vi "lj_read.vi"(7 "Queues":T1, 8 "error in (no error)":errorcluster, 11 "LabJackConfig":T4={"Drum Reflectors"=4, "Drum Max. Samping Window [s]"=2.0, "Drum Min. Sampling Window [s]"=0.5, "Flow Max. Samping Window [s]"=1.0, "Flow Min. Sampling Window [s]"=0.25, "Pulse value [mL]"=0.0, "RMS Sampling Window [s]"=3.0, "TC Sampling Window [s]"=0.25, "TC Scale"=[1.0, 1.0], "TC Offset [V]"=[0.0, 0.0]} {"TC Offset [V]" format="%#_f"; "TC Scale" format="%#_f"; "Pulse value [mL]" format="%#_f"}) -> (0 "error out":errorcluster, 2 "subarray":dbl[](array[numeric]), 3 "Read Data":T3 {"Peak to Peak [V]" format="%#_f"; "RMS [Hz]" format="%#_f"; "CJTemp [K]" format="%#_f"; "TC [V]" format="%#_f"; "TC [degC]" format="%#_f"; "RMS [A]" format="%#_f"; "Volume [L]" format="%#_f"; "Flow [L/min]" format="%#_f"; "Spin  [RPM]" format="%#_f"})   [LabVIEW 2025, in "LabJackEKG.lvlib"]
uses:
  LabJackEKG.lvlib
  Typedefs/AcquisitionConfig.ctl
  Typedefs/LabJackData.ctl
  Typedefs/LabJackGlobalResources.ctl
  Typedefs/CounterQueues.ctl
  Typedefs/DirectionFgvOperation.ctl
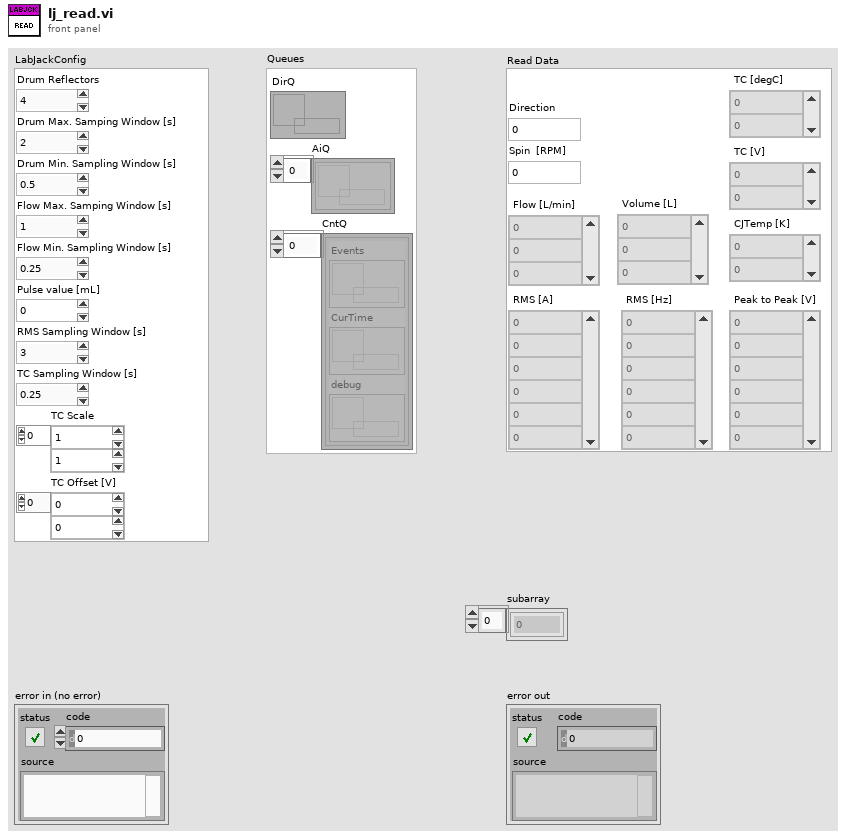
[diagram p1: front panel]
types:
  T1 = typedef "LabJackEKG.lvlib/LabJackGlobalResources.ctl" = cluster{"DirQ":refnum<queue>, "AiQ":refnum<queue>[], "CntQ":T2[]}
  T2 = typedef "LabJackEKG.lvlib/CounterQueues.ctl" = cluster{"Events":refnum<queue>, "CurTime":refnum<queue>, "debug":refnum<queue>}
  T3 = typedef "LabJackEKG.lvlib/LabJackData.ctl" = cluster{"Direction":i32, "Spin  [RPM]":dbl, "Flow [L/min]":dbl[], "Volume [L]":dbl[], "RMS [A]":dbl[], "TC [degC]":dbl[], "TC [V]":dbl[], "CJTemp [K]":dbl[], "RMS [Hz]":dbl[], "Peak to Peak [V]":dbl[]}
  T4 = typedef "LabJackEKG.lvlib/AcquisitionConfig.ctl" = cluster{"Drum Reflectors":i64, "Drum Max. Samping Window [s]":dbl, "Drum Min. Sampling Window [s]":dbl, "Flow Max. Samping Window [s]":dbl, "Flow Min. Sampling Window [s]":dbl, "Pulse value [mL]":dbl, "RMS Sampling Window [s]":dbl, "TC Sampling Window [s]":dbl, "TC Scale":dbl[], "TC Offset [V]":dbl[]}
  T5 = typedef "LabJackEKG.lvlib/DirectionFgvOperation.ctl" = enum16{"init", "process", "get"}
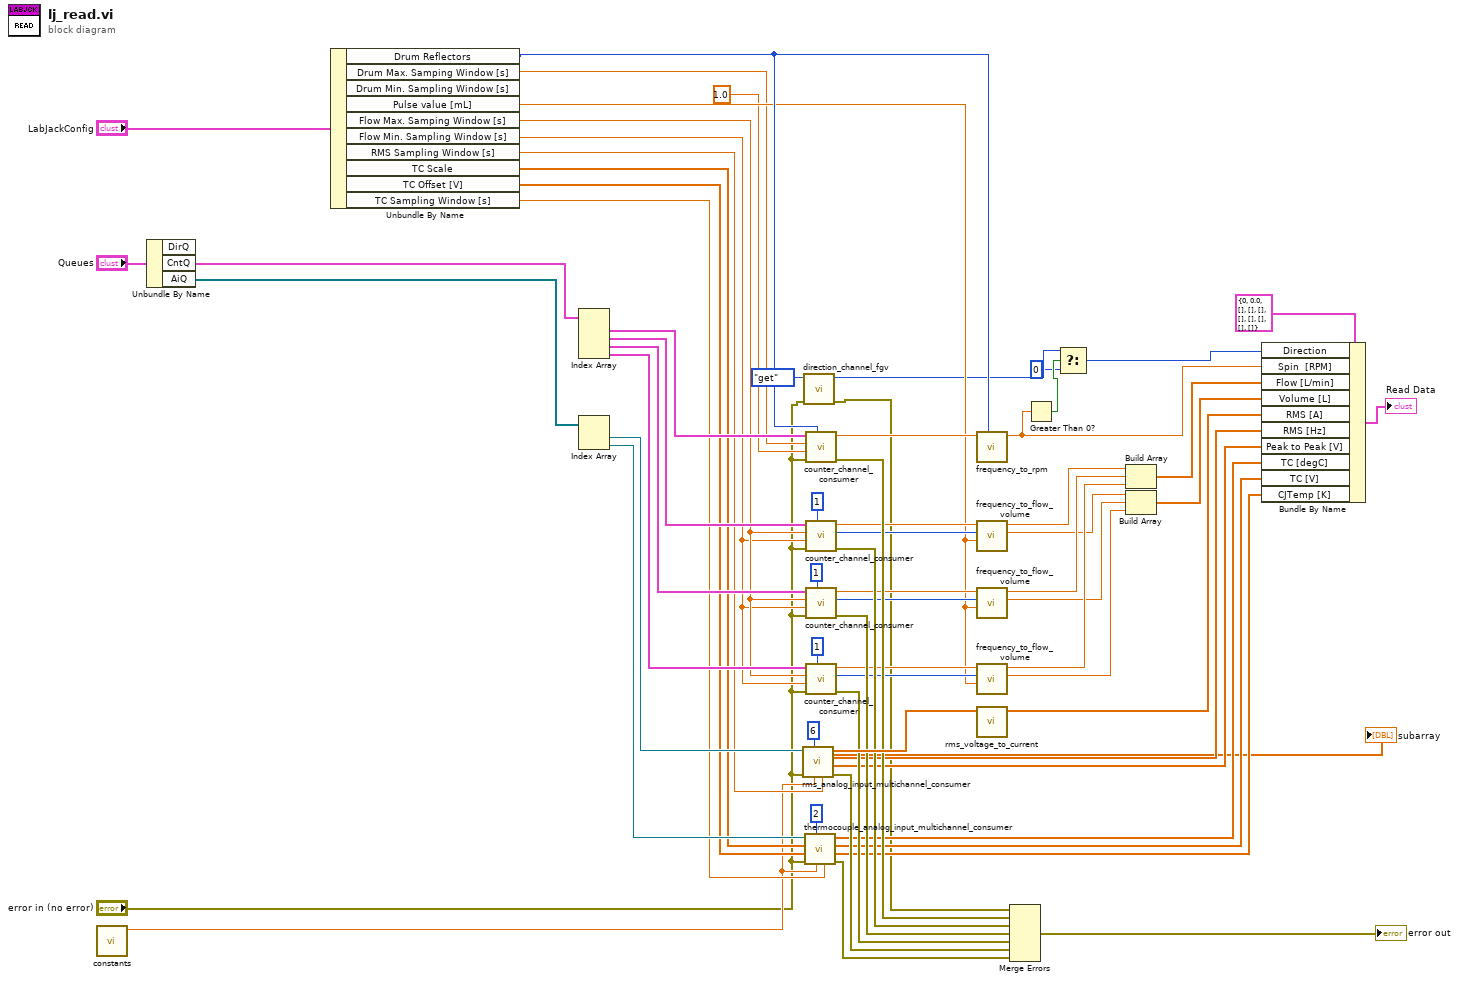
[diagram p0: block diagram]
diagram:
  n1 = call "constants.vi"() -> ("Sampling Frequency [Hz]"=w11:dbl)  [unwired: 10 in, 1 out]
  n2 = Unbundle By Name("Queues") -> ("CntQ"=w19:T2[], "AiQ"=w18:refnum<queue>[])  [unwired: 1 out]
  n3 = Unbundle By Name("LabJackConfig") -> ("Drum Reflectors"=w38:i64, "Drum Max. Samping Window [s]"=w10:dbl, "Pulse value [mL]"=w15:dbl, "Flow Max. Samping Window [s]"=w45:dbl, "Flow Min. Sampling Window [s]"=w44:dbl, "RMS Sampling Window [s]"=w43:dbl, "TC Scale"=w42:dbl[], "TC Offset [V]"=w41:dbl[], "TC Sampling Window [s]"=w40:dbl)  [unwired: 1 out]
  n4 = Index Array(array=w19) -> (element #1=w63:T2, element #2=w62:T2, element #3=w61:T2, element #4=w60:T2)  [unwired: 4 in]
  n5 = Index Array(array=w18) -> (element #1=w54:refnum<queue>, element #2=w55:refnum<queue>)  [unwired: 2 in]
  n6 = call "rms_analog_input_multichannel_consumer.vi"("Sampling Window [s]"=w43, "Sampling Frequency [Hz]"=w11, "Number of Channels"=6, "error in (no error)"="error in (no error)", "queue out"=w54) -> ("error out"=w51:errorcluster, "Peak to Peak [V]"=w13:dbl[], "Detected  [Hz]"=w14:dbl[], "RMS [V]"=w53:dbl[], "subarray"=→"subarray":dbl[])  [unwired: 2 in]
  n7 = call "direction_channel_fgv.vi"("error in (no error)"="error in (no error)", "op"=DirectionFgvOperation."get") -> ("error out"=w8:errorcluster, "direction"=w5:i64)  [unwired: 8 in]
  n8 = call "thermocouple_analog_input_multichannel_consumer.vi"("Sampling Window [s]"=w40, "Sampling Frequency [Hz]"=w11, "Number of Channels"=2, "error in (no error)"="error in (no error)", "Offset [V]"=w41, "Scale"=w42, "queue out"=w55) -> ("error out"=w52:errorcluster, "CJTemp[K]"=w16:dbl[], "TC [V]"=w17:dbl[], "TC [degC]"=w21:dbl[])  [unwired: 1 in]
  n9 = call "counter_channel_consumer.vi"("Sample Group Size"=w38, "error in (no error)"="error in (no error)", "Min. Sampling Window [s]"=1.0, "Max. Samping Window [s]"=w10, "Queue in"=w63) -> ("error out"=w47:errorcluster, "Pulse Frequency [Hz]"=w39:dbl)  [unwired: 2 in, 3 out]
  n10 = call "counter_channel_consumer.vi"("Sample Group Size"=i64 1, "error in (no error)"="error in (no error)", "Min. Sampling Window [s]"=w44, "Max. Samping Window [s]"=w45, "Queue in"=w62) -> ("error out"=w48:errorcluster, "Pulse Count"=w34:i64, "Pulse Frequency [Hz]"=w35:dbl)  [unwired: 2 in, 2 out]
  n11 = call "counter_channel_consumer.vi"("Sample Group Size"=i64 1, "error in (no error)"="error in (no error)", "Min. Sampling Window [s]"=w44, "Max. Samping Window [s]"=w45, "Queue in"=w61) -> ("error out"=w49:errorcluster, "Pulse Count"=w33:i64, "Pulse Frequency [Hz]"=w37:dbl)  [unwired: 2 in, 2 out]
  n12 = call "counter_channel_consumer.vi"("Sample Group Size"=i64 1, "error in (no error)"="error in (no error)", "Min. Sampling Window [s]"=w44, "Max. Samping Window [s]"=w45, "Queue in"=w60) -> ("error out"=w50:errorcluster, "Pulse Count"=w32:i64, "Pulse Frequency [Hz]"=w36:dbl)  [unwired: 2 in, 2 out]
  n13 = call "frequency_to_rpm.vi"("Number of Stickers"=w38, "Pulse Frequency [Hz]"=w39) -> ("Spin [RPM]"=w3:dbl)  [unwired: 9 in]
  n14 = call "frequency_to_flow_volume.vi"("mlL/pulse"=w15, "Pulse Count"=w34, "Pulse Frequency [Hz]"=w35) -> ("Volume [L]"=w28:dbl, "Flow [L/min]"=w31:dbl)  [unwired: 7 in]
  n15 = call "frequency_to_flow_volume.vi"("mlL/pulse"=w15, "Pulse Count"=w33, "Pulse Frequency [Hz]"=w37) -> ("Volume [L]"=w27:dbl, "Flow [L/min]"=w30:dbl)  [unwired: 7 in]
  n16 = call "frequency_to_flow_volume.vi"("mlL/pulse"=w15, "Pulse Count"=w32, "Pulse Frequency [Hz]"=w36) -> ("Volume [L]"=w26:dbl, "Flow [L/min]"=w29:dbl)  [unwired: 7 in]
  n17 = call "rms_voltage_to_current.vi"("RMS [V]"=w53) -> ("RMS[A]"=w22:dbl[])  [unwired: 10 in]
  n18 = Merge Errors(w8, w47, w48, w49, w50, w51, w52) -> (→"error out":errorcluster)
  n19 = Greater Than 0?(x=w3) -> (x > 0?=w2:bool)
  n20 = Select(t=w5, s=w2, f=i64 0) -> (s? t:f=w4:i64)
  n21 = Build Array(w31, w30, w29) -> (w24:dbl[])
  n22 = Build Array(w28, w27, w26) -> (w23:dbl[])
  n23 = Bundle By Name(cluster=T3 {"Direction"=0, "Spin  [RPM]"=0.0, "Flow [L/min]"=[], "Volume [L]"=[], "RMS [A]"=[], "TC [degC]"=[], "TC [V]"=[], "CJTemp [K]"=[], "RMS [Hz]"=[], "Peak to Peak [V]"=[]} ("LabJack Data"), "Direction"=w4, "Spin  [RPM]"=w3, "Flow [L/min]"=w24, "Volume [L]"=w23, "RMS [A]"=w22, "RMS [Hz]"=w14, "Peak to Peak [V]"=w13, "TC [degC]"=w21, "TC [V]"=w17, "CJTemp [K]"=w16) -> (→"Read Data":T3)
